vi "Display_data.vi"() -> (0 "STOP ALL 2":bool)   [LabVIEW 2016]
uses:
  <vilib>/Utility/file.llb/Read Delimited Spreadsheet (DBL).vi
panel:
  in  "Boolean":bool
  in  "STOP ALL":bool
  in  "stop":bool
  in  "Ring":u16(ring) items=["Default", "Number Filter", "Average", "Integrate", "Derivate", "g"]
  in  "String":string
  out "Waveform Graph 2":dbl[](graph)
  out "Array":dbl[](array[numeric])
  in  "X vector":i32
  out "XY Graph":cluster{dbl[], "all rows":dbl[]}[](graph)
  in  "Inoput":dbl=15.0 format="%#_13g"
  in  "index (row) 3":i32
  in  "index (row) 2":i32
  in  "index (row)":i32
  out "all rows":dbl[][](array[numeric])
  out "Raw Data":dynamicdata(graph)
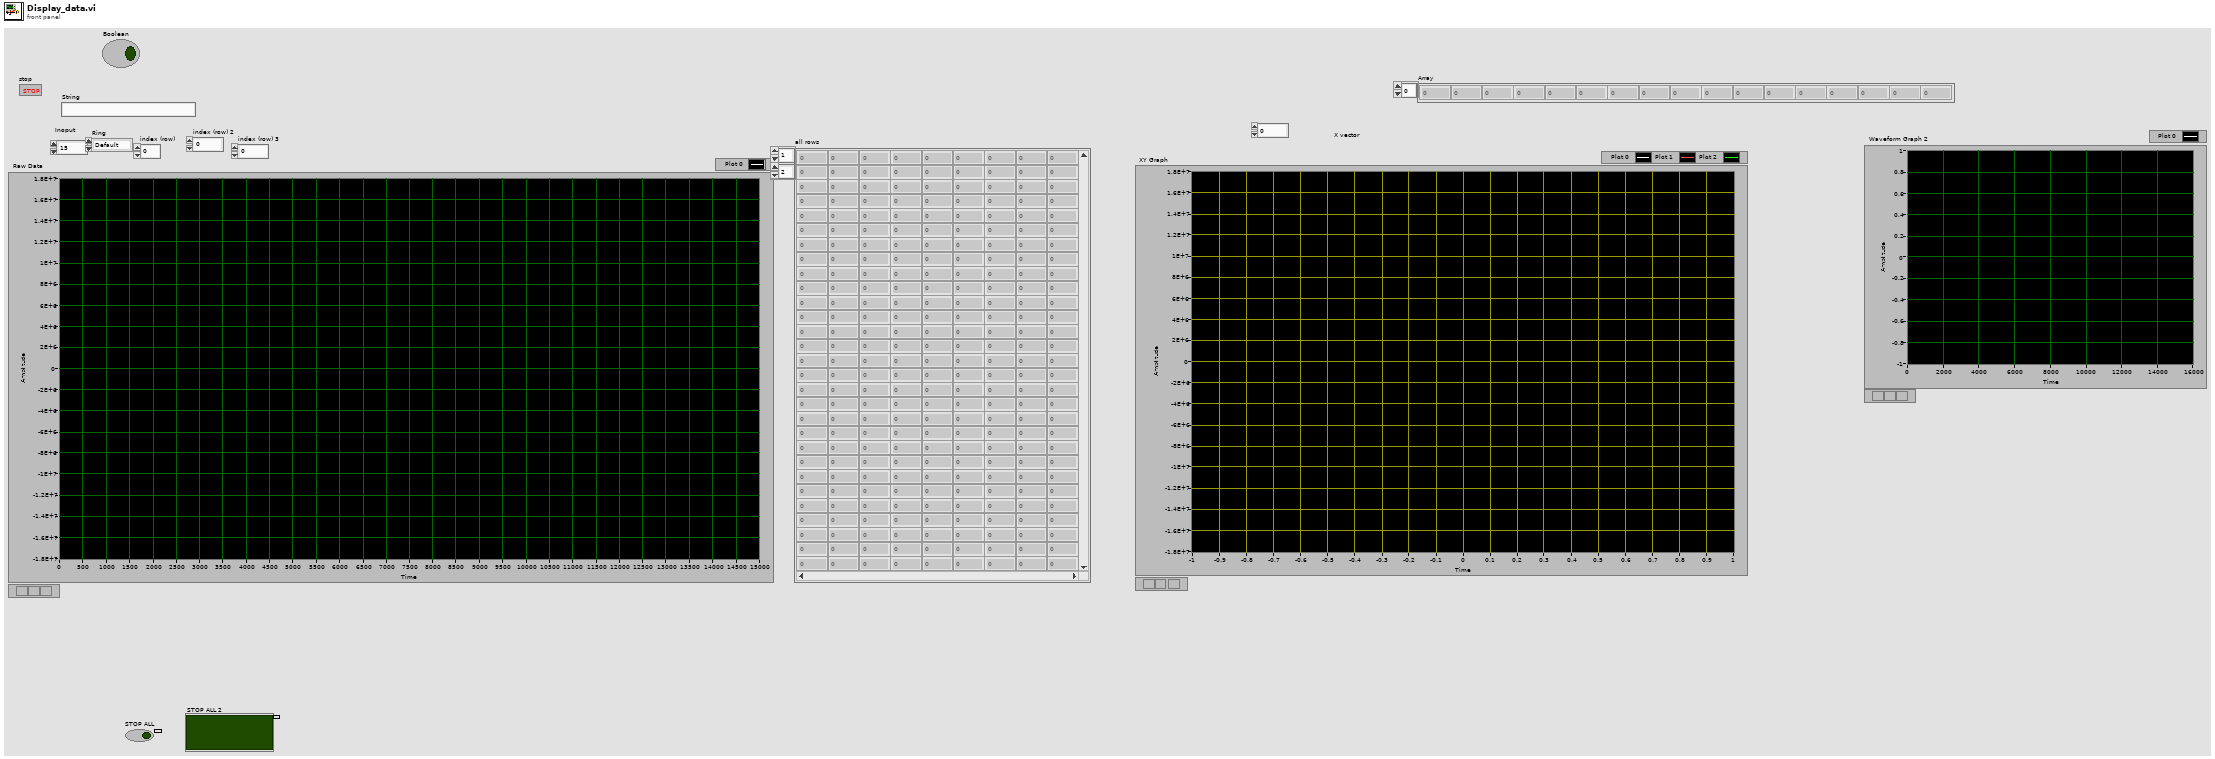
[diagram p1: front panel]
types:
  T1 = cluster{"Output Array":dbl[], "Output Array":dbl[]}
  T2 = cluster{"Output Array":dbl[], "Output Array":dbl[]}[]
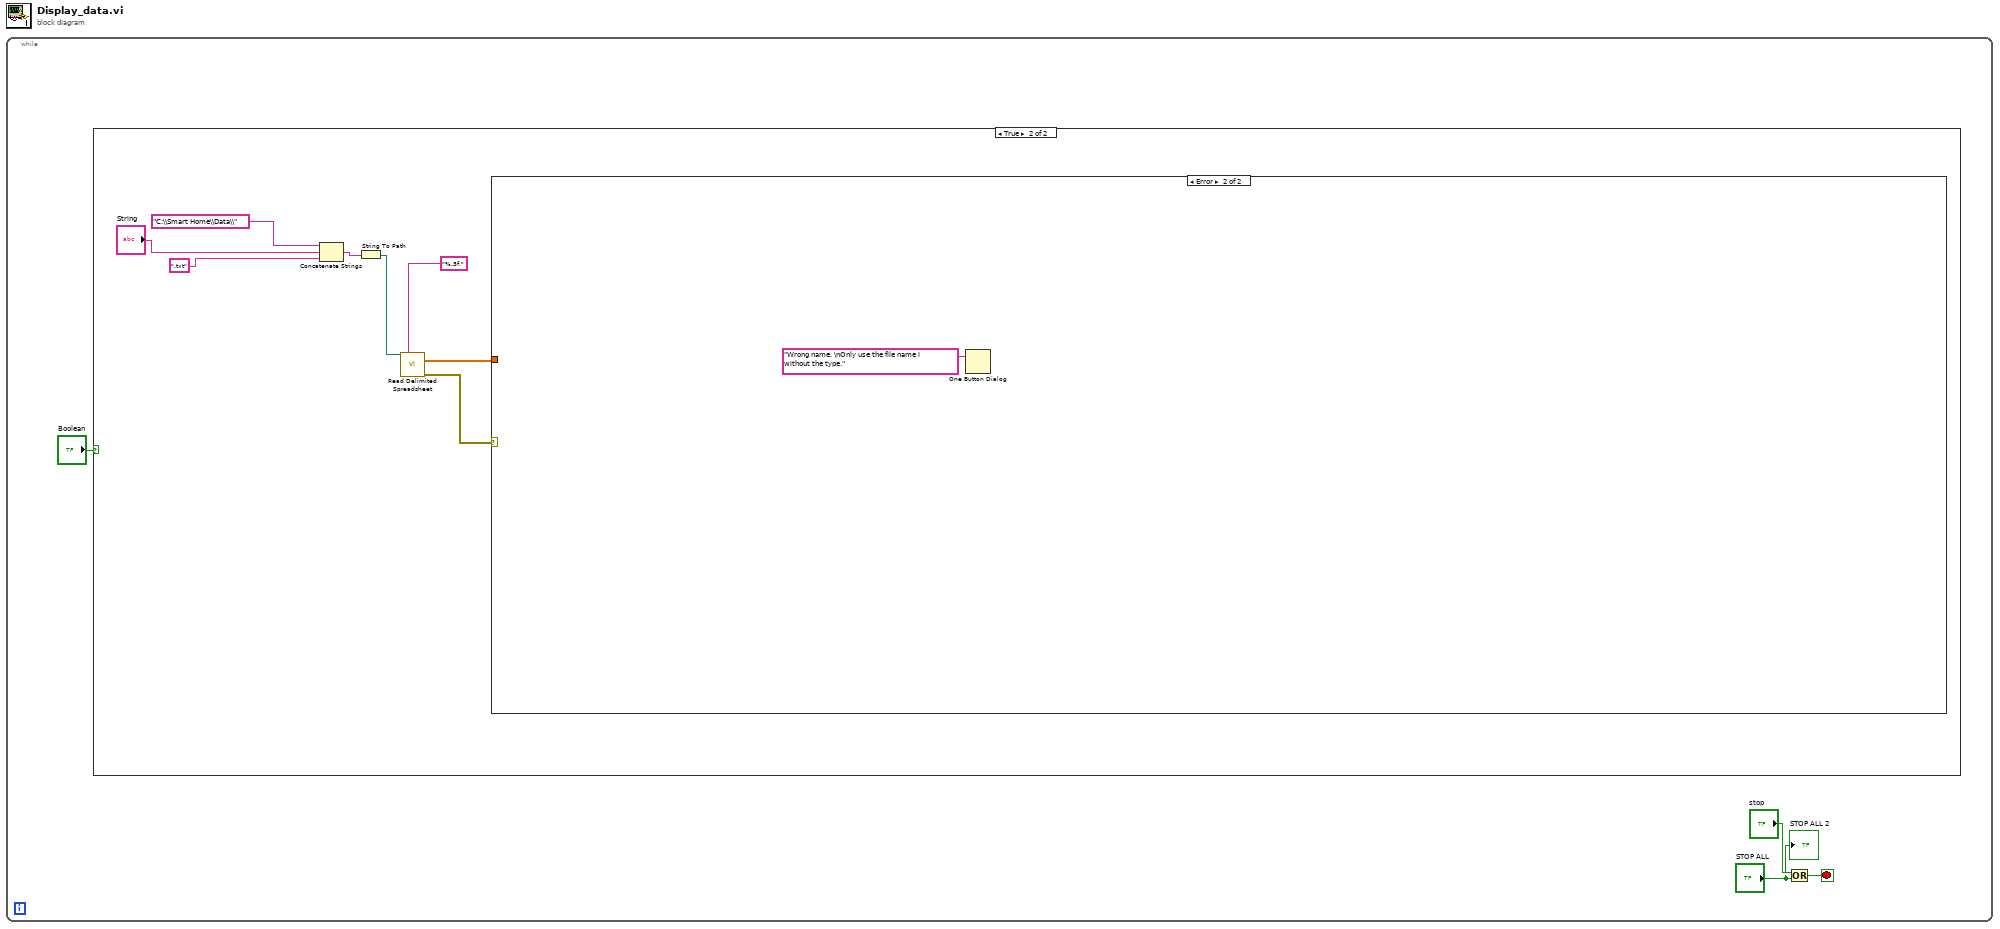
[diagram p0: block diagram]
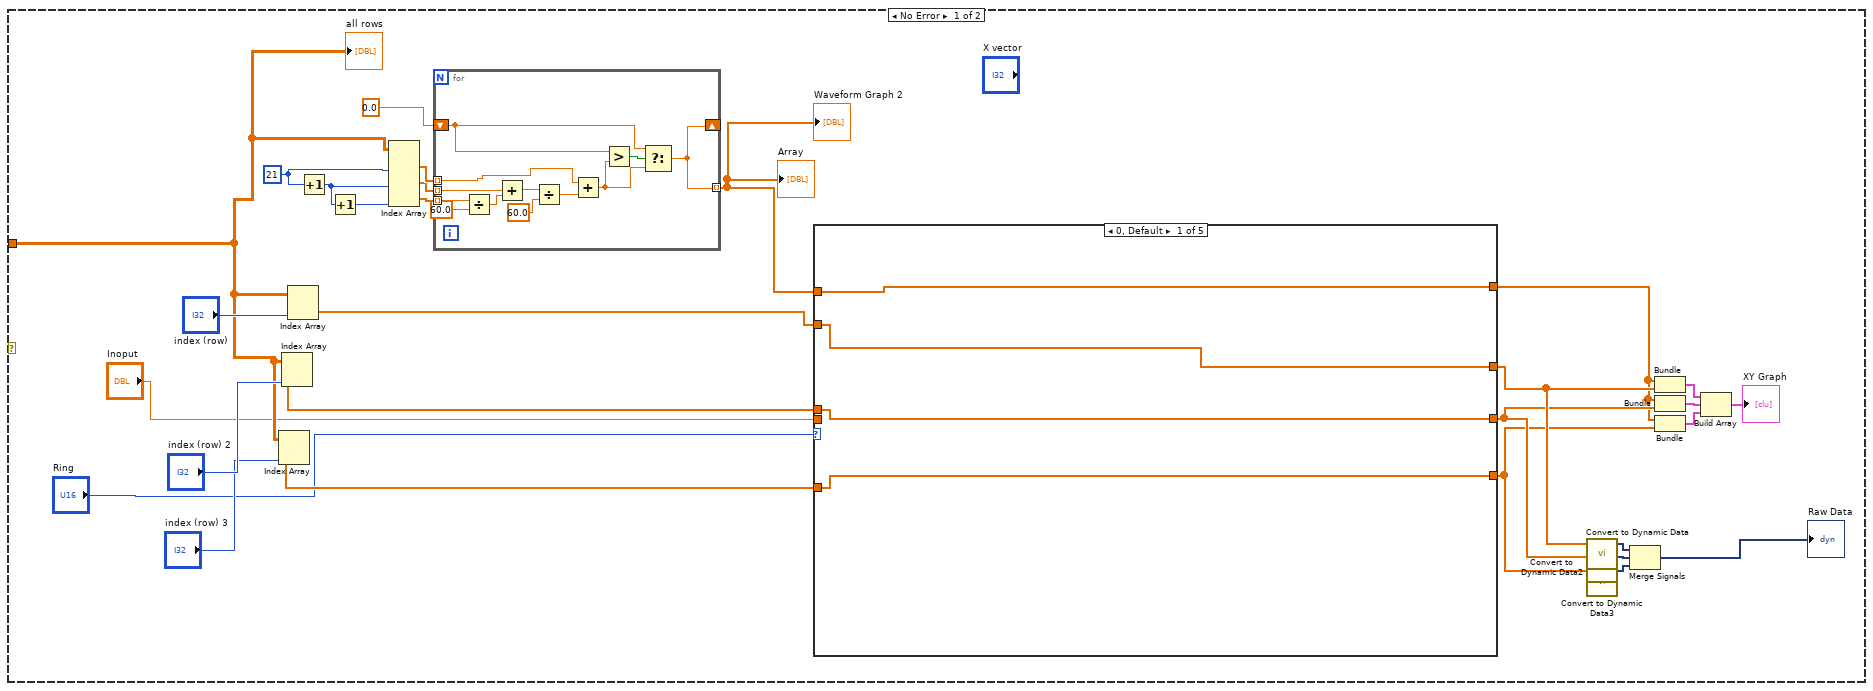
[diagram p3: hidden frame]
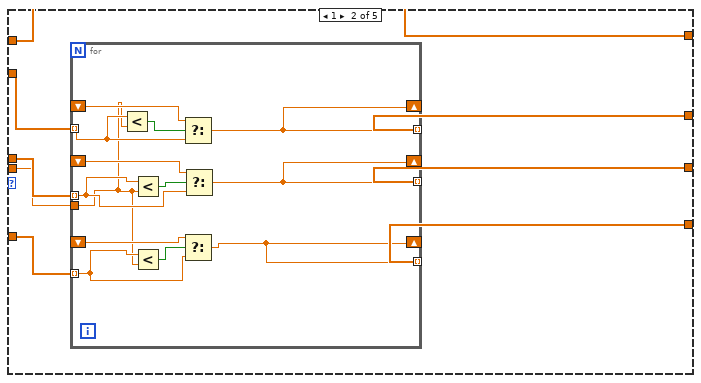
[diagram p4: hidden frame]
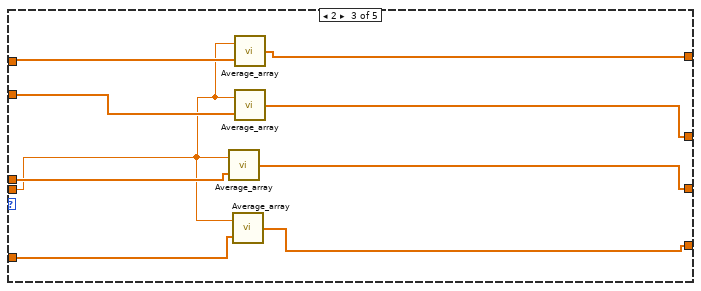
[diagram p5: hidden frame]
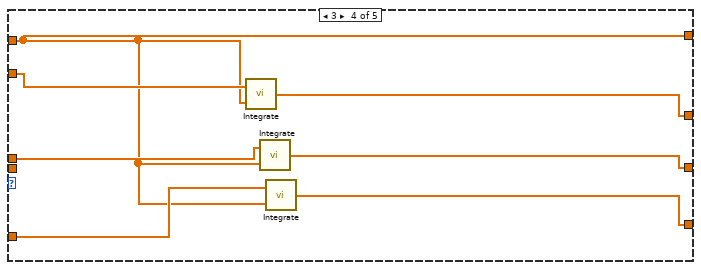
[diagram p6: hidden frame]
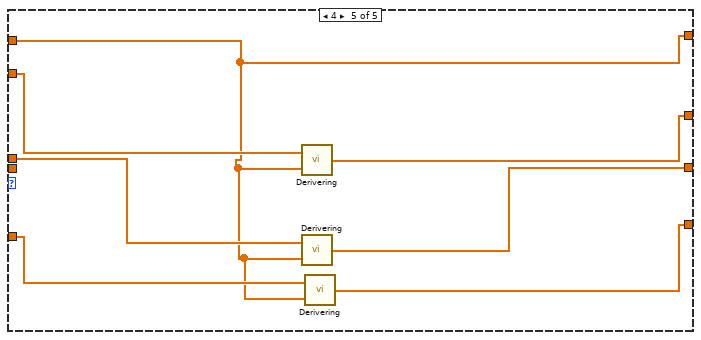
[diagram p7: hidden frame]
diagram:
  n1 = while {
    stop <- w3 stop-if-true
    n2 = case shown="True" "Boolean" {
      frame False {
      }
      frame True {
        n3 = Concatenate Strings("C:\\Smart Home\\Data\\", "String", ".txt") -> (w10:string)
        n4 = String To Path(string=w10) -> (path=w6:path)
        n5 = call-poly <vilib>:"Read Delimited Spreadsheet.vi"("file path (dialog if empty)"=w6, "format (%.3f)"="%.3f,") -> ("all rows"=w11:dbl[][], "error out"=w5:errorcluster)  [unwired: 8 in, 4 out]
        n6 = case shown="Error" w5 {
          tunnel: w11 -> [w31 _]
          frame No Error {
            w30 = 21 ("index (col)")
            n7 = Index Array(array=w31, index (col)="index (row) 3") -> (element=w32:dbl[])  [unwired: 1 in]
            n8 = Index Array(array=w31, index (col)="index (row) 2") -> (element=w33:dbl[])  [unwired: 1 in]
            n9 = Index Array(array=w31, index (col)="index (row)") -> (element=w34:dbl[])  [unwired: 1 in]
            n10 = Increment(x=w30) -> (x+1=w25:i32)
            n11 = Increment(x=w25) -> (x+1=w29:i32)
            n12 = Index Array(array=w31, index (col) #1=w30, index (col) #2=w25, index (col) #3=w29) -> (element #1=w28:dbl[], element #2=w27:dbl[], element #3=w26:dbl[])  [unwired: 3 in]
            n13 = for {
              tunnel: w28 -> [w45] mode=indexing
              tunnel: w27 -> [w47] mode=indexing
              tunnel: w26 -> [w46] mode=indexing
              tunnel: [w44] -> w14 mode=indexing
              shift-right: [w44] -> _
              shift-left: 0.0 -> [w43]
              n14 = Divide(x=w46, y=60.0) -> (x/y=w53:dbl)
              n15 = Add(x=w47, y=w53) -> (x+y=w48:dbl)
              n16 = Divide(x=w48, y=60.0) -> (x/y=w52:dbl)
              n17 = Add(x=w45, y=w52) -> (x+y=w42:dbl)
              n18 = Greater?(x=w43, y=w42) -> (0:w49:bool)
              n19 = Select(t=w43, s=w49, f=w42) -> (s? t:f=w44:dbl)
            }
            "Array" <- w14
            "Waveform Graph 2" <- w14
            n20 = case shown="0, Default" "Ring" {
              tunnel: w34 -> [w57 w65 w85 w92 w101]
              tunnel: w33 -> [w56 w64 w86 w93 w100]
              tunnel: w32 -> [w55 w63 w87 w94 w99]
              tunnel: [w55 w62 w82 w89 w98] -> w21
              tunnel: [w56 w61 w83 w90 w97] -> w22
              tunnel: [w57 w60 w84 w91 w96] -> w24
              tunnel: "Inoput" -> [_ w59 w80 _ _]
              tunnel: w14 -> [w54 w58 w81 w88 w95]
              tunnel: [w54 w58 w79 w88 w95] -> w13
              frame 0, Default {
              }
              frame 1 {
                n21 = for {
                  tunnel: w65 -> [w76] mode=indexing
                  tunnel: w64 -> [w73] mode=indexing
                  tunnel: w63 -> [w70] mode=indexing
                  shift-right: [w67] -> _
                  shift-left: _ -> [w68]
                  shift-right: [w72] -> _
                  shift-left: _ -> [w71]
                  shift-right: [w78] -> _
                  shift-left: _ -> [w77]
                  tunnel: [w78] -> w60 mode=indexing
                  tunnel: [w72] -> w61 mode=indexing
                  tunnel: [w67] -> w62 mode=indexing
                  tunnel: w59 -> [w66]
                  n22 = Less?(x=w76, y=w66) -> (x < y?=w75:bool)
                  n23 = Less?(x=w73, y=w66) -> (x < y?=w74:bool)
                  n24 = Less?(x=w70, y=w66) -> (x < y?=w69:bool)
                  n25 = Select(t=w77, s=w75, f=w76) -> (s? t:f=w78:dbl)
                  n26 = Select(t=w68, s=w69, f=w70) -> (s? t:f=w67:dbl)
                  n27 = Select(t=w71, s=w74, f=w73) -> (s? t:f=w72:dbl)
                }
              }
              frame 2 {
                n28 = call "Average_array.vi"("Input Array"=w86, "Average over.."=w80) -> ("Output Array"=w83:dbl[])
                n29 = call "Average_array.vi"("Input Array"=w87, "Average over.."=w80) -> ("Output Array"=w82:dbl[])
                n30 = call "Average_array.vi"("Input Array"=w81, "Average over.."=w80) -> ("Output Array"=w79:dbl[])
                n31 = call "Average_array.vi"("Input Array"=w85, "Average over.."=w80) -> ("Output Array"=w84:dbl[])
              }
              frame 3 {
                n32 = call "Integrate.vi"("Input Array Y"=w88, "Input Array X"=w92) -> ("Output Array"=w91:dbl[])
                n33 = call "Integrate.vi"("Input Array Y"=w88, "Input Array X"=w93) -> ("Output Array"=w90:dbl[])
                n34 = call "Integrate.vi"("Input Array Y"=w88, "Input Array X"=w94) -> ("Output Array"=w89:dbl[])
              }
              frame 4 {
                n35 = call "Derivering.vi"("Input Array Y"=w95, "Input Array X"=w101) -> ("Output Array"=w96:dbl[])
                n36 = call "Derivering.vi"("Input Array Y"=w95, "Input Array X"=w100) -> ("Output Array"=w97:dbl[])
                n37 = call "Derivering.vi"("Input Array Y"=w95, "Input Array X"=w99) -> ("Output Array"=w98:dbl[])
              }
            }
            n38 = call "Convert to Dynamic Data"("Array"=w24) -> ("Dynamic Data Type"=w38:dynamicdata)  [unwired: 3 in]
            n39 = call "Convert to Dynamic Data2"("Array"=w22) -> ("Dynamic Data Type"=w37:dynamicdata)  [unwired: 3 in]
            n40 = call "Convert to Dynamic Data3"("Array"=w21) -> ("Dynamic Data Type"=w36:dynamicdata)  [unwired: 3 in]
            n41 = Merge Signals(w38, w37, w36) -> (→"Raw Data":dynamicdata)
            n42 = Bundle("Output Array"=w13, "Output Array"=w24) -> (w20:T1)  [unwired: 1 in]
            n43 = Bundle("Output Array"=w13, "Output Array"=w22) -> (w19:T1)  [unwired: 1 in]
            n44 = Bundle("Output Array"=w13, "Output Array"=w21) -> (w18:T1)  [unwired: 1 in]
            n45 = Build Array(w20, w19, w18) -> (→"XY Graph":T2)
            "all rows" <- w31
          }
          frame Error {
            n46 = One Button Dialog(message="Wrong name. \nOnly use the file name i without the type.") -> ()  [unwired: 1 in, 1 out]
          }
        }
      }
    }
    n47 = Or(x="stop", y="STOP ALL") -> (x .or. y?=w3:bool)
    "STOP ALL 2" <- "STOP ALL"
  }
